vi "ADIS16470 Decode AutoSPI.vi"(8 "error in (no error)":errorcluster, 9 "TimeStampPrev":u32, 10 "Bytes Per Sample":u32, 11 "Data in":dbl[](array[numeric])) -> (0 "error out":errorcluster, 2 "Last Timestamp":u32, 3 "Data out":dbl[](array[numeric]), 5 "Raw Data":cluster{"Theta":dbl[], "Timestamp":u32}[](array[cluster]))   [LabVIEW 2019]
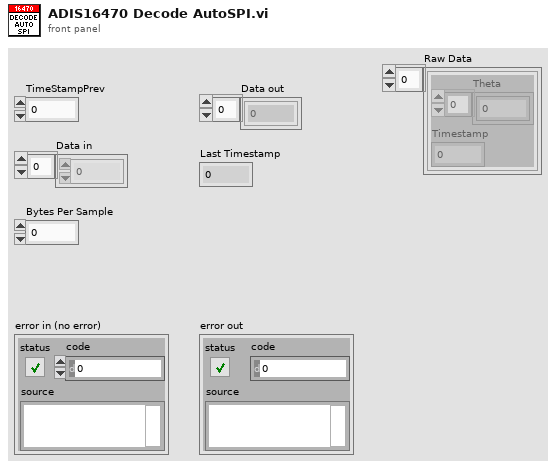
[diagram p1: front panel]
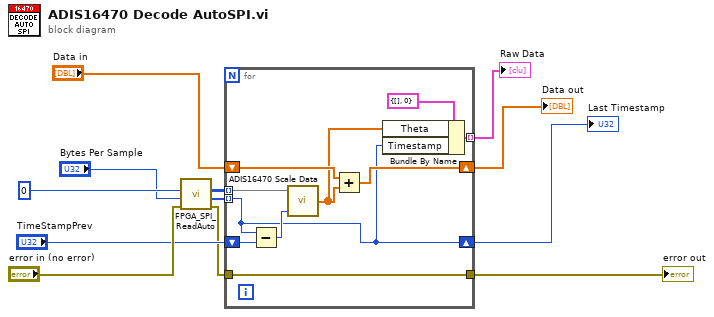
[diagram p0: block diagram]
diagram:
  n1 = call <vilib>:"FPGA_SPI_ReadAuto.vi"("error in (no error)"="error in (no error)", "Bytes per Sample"="Bytes Per Sample", "Samples to Read"=u32 0) -> ("error out"=w8:errorcluster, "Timestamps"=w6:u32[], "Data"=w5:u8[][])  [unwired: 5 in, 1 out]
  n2 = for {
    tunnel: w5 -> [w19] mode=indexing
    tunnel: w6 -> [w15] mode=indexing
    shift-right: [w16] -> w2
    shift-left: "Data in" -> [w22]
    tunnel: w8 -> [w20]
    tunnel: [w20] -> w9
    shift-right: [w15] -> w11
    shift-left: "TimeStampPrev" -> [w21]
    tunnel: [w14] -> w1 mode=indexing
    n3 = Subtract(x=w15, y=w21) -> (x-y=w18:u32)
    n4 = call "ADIS16470 Scale Data.vi"("TimeStamp"=w18, "Data In"=w19) -> ("Scaled Data Out"=w13:dbl[])  [unwired: 3 in]
    n5 = Add(x=w22, y=w13) -> (x+y=w16:dbl[])
    n6 = Bundle By Name(cluster=cluster{"Theta":dbl[], "Timestamp":u32} {"Theta"=[], "Timestamp"=0}, "Theta"=w13, "Timestamp"=w15) -> (w14:cluster{"Theta":dbl[], "Timestamp":u32})
  }
  "Last Timestamp" <- w11
  "error out" <- w9
  "Data out" <- w2
  "Raw Data" <- w1
